vi "Get VS Channel Handles and Messages.vi"(8 "error in":errorcluster, 11 "custom device ref":T2 format="%.0x") -> (0 "error out":errorcluster, 1 "outgoing channels":T2[](array[typedef]) format="%.0x", 2 "incoming channels":T2[](array[typedef]) format="%.0x", 3 "custom device ref out":T2 format="%.0x", 4 "transmitted messages and subaddresses":T1[](array[typedef]) {"Timestamp Channel Handle" format="%.0x"; "Message Section Handle" format="%.0x"; "Parameter Channel Handles" format="%.0x"}, 6 "received messages and subaddresses":T1[](array[typedef]) {"Timestamp Channel Handle" format="%.0x"; "Message Section Handle" format="%.0x"; "Parameter Channel Handles" format="%.0x"})   [LabVIEW 2020, in "AIM MIL-STD-1553 Engine.lvlib" / "Implementation.lvlib" / "Execution Unit.lvclass"]
uses:
  Execution Unit.lvclass
  <vilib>/NI VeriStand/Custom Device API/Custom Device Item Ref.ctl
  Custom Device/Compiled Message.ctl
  Shared/Direction.ctl
  Shared/Parameter Definition.ctl
  <vilib>/NI VeriStand/Custom Device API/Custom Device API.lvlib
  Scripting/AIM MIL-STD-1553 Scripting.lvlib
  Custom Device/Custom Device.lvlib
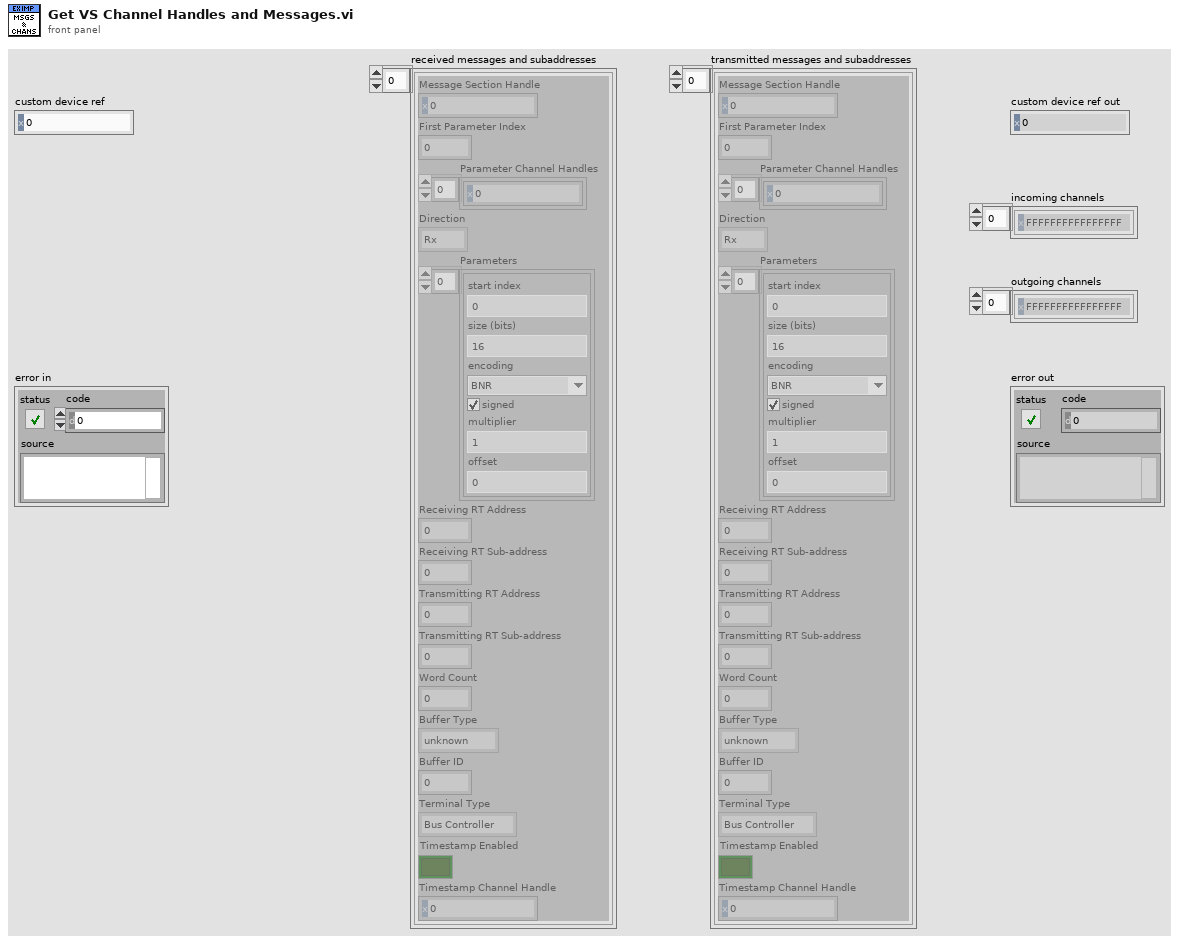
[diagram p1: front panel]
types:
  T1 = typedef "AIM MIL-STD-1553 Engine.lvlib/Custom Device.lvlib/Compiled Message.ctl" = cluster{"Message Section Handle":T2, "First Parameter Index":i32, "Parameter Channel Handles":T2[], "Direction":T3, "Parameters":T4[], "Receiving RT Address":u8, "Receiving RT Sub-address":u8, "Transmitting RT Address":u8, "Transmitting RT Sub-address":u8, "Word Count":u8, "Buffer Type":enum16{"unknown", "BC Message Buffer", "RT Message Buffer"}, "Buffer ID":u16, "Terminal Type":enum16{"Bus Controller", "Remote Terminal"}, "Timestamp Enabled":bool, "Timestamp Channel Handle":T2}
  T2 = typedef "Custom Device API.lvlib/Custom Device Item Ref.ctl" = u64
  T3 = typedef "Direction.ctl" = enum16{"Rx", "Tx"}
  T4 = typedef "Parameter Definition.ctl" = cluster{"start index":i32, "size (bits)":i32, "encoding":enum16{"BNR", "BCD", "Discrete"}, "signed":bool, "multiplier":dbl, "offset":dbl}
  T5 = typedef "Terminal Endpoint.ctl" = cluster{"terminal address":T6, "subaddress":T6}
  T6 = typedef "Address.ctl" = u16
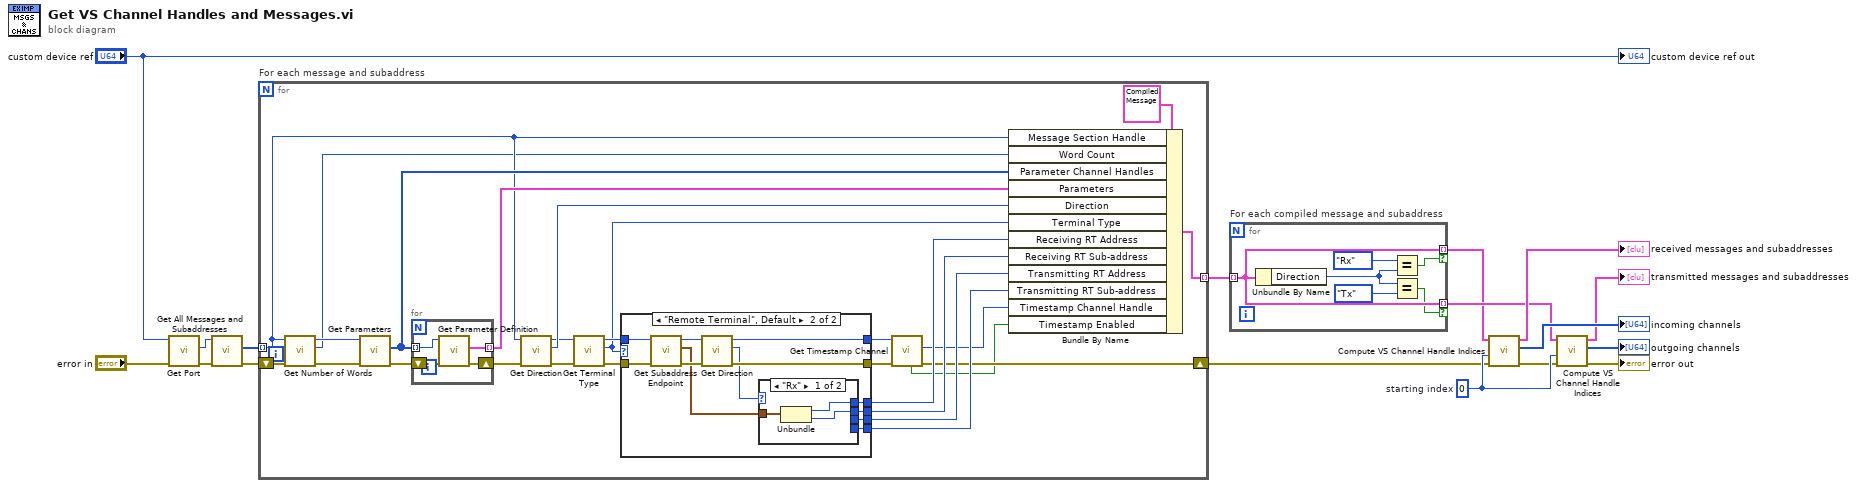
[diagram p0: block diagram]
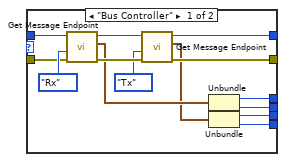
[diagram p2: hidden frame]
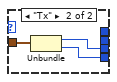
[diagram p3: hidden frame]
diagram:
  w12 = 0  # starting index
  n1 = call "Get Port.vi"("error in"="error in", "custom device ref"="custom device ref") -> ("error out"=w4:errorcluster, "port"=w3:T2)  [unwired: 6 in, 2 out]
  n2 = call "Get All Messages and Subaddresses.vi"("error in"=w4, "port"=w3) -> ("error out"=w11:errorcluster, "messages and subaddresses"=w10:T2[])  [unwired: 7 in, 1 out]
  n3 = for "For each message and subaddress" {
    shift-right: [w21] -> w6
    shift-left: w11 -> [w27]
    tunnel: w10 -> [w28] mode=indexing
    tunnel: [w43] -> w9 mode=indexing
    n4 = call "Get Number of Words.vi"("error in"=w27, "message or subaddress"=w28) -> ("error out"=w26:errorcluster, "number of words"=w24:u16, "message or subaddress out"=w25:T2)  [unwired: 7 in]
    n5 = call "Get Parameters.vi"("error in"=w26, "message or subaddress"=w25) -> ("error out"=w40:errorcluster, "parameters"=w39:T2[])  [unwired: 7 in, 1 out]
    n6 = for {
      shift-right: [w79] -> w37
      shift-left: w40 -> [w78]
      tunnel: w39 -> [w77] mode=indexing
      tunnel: [w76] -> w38 mode=indexing
      n7 = call "Get Parameter Definition.vi"("error in"=w78, "parameter"=w77) -> ("error out"=w79:errorcluster, "parameter definition"=w76:T4)  [unwired: 7 in, 1 out]
    }
    n8 = call "Get Direction.vi"("error in"=w37, "message or subaddress"=w28) -> ("error out"=w34:errorcluster, "direction"=w41:T3, "message or subaddress out"=w33:T2)  [unwired: 6 in, 1 out]
    n9 = call "Get Terminal Type.vi"("error in"=w34, "message or subaddress"=w33) -> ("error out"=w36:errorcluster, "terminal type"=w23:enum16{"Bus Controller", "Remote Terminal"}, "message or subaddress out"=w35:T2)  [unwired: 7 in]
    n10 = case shown="\"Remote Terminal\", Default" w23 {
      tunnel: [w51 w67] -> w20
      tunnel: [w50 w66] -> w22
      tunnel: w35 -> [w57 w63]
      tunnel: w36 -> [w55 w62]
      tunnel: [w44 w61] -> w29
      tunnel: [w45 w60] -> w30
      tunnel: [w48 w59] -> w31
      tunnel: [w49 w58] -> w32
      frame "Bus Controller" {
        n11 = call "Get Message Endpoint.vi"("error in"=w55, "direction"=Direction."Rx", "message"=w57) -> ("error out"=w54:errorcluster, "remote terminal endpoint"=w47:T5, "message out"=w52:T2)  [unwired: 5 in, 1 out]
        n12 = call "Get Message Endpoint.vi"("error in"=w54, "direction"=Direction."Tx", "message"=w52) -> ("error out"=w50:errorcluster, "remote terminal endpoint"=w46:T5, "message out"=w51:T2)  [unwired: 5 in, 1 out]
        n13 = Unbundle(w47) -> ("terminal address"=w49:T6, "subaddress"=w48:T6)
        n14 = Unbundle(w46) -> ("terminal address"=w45:T6, "subaddress"=w44:T6)
      }
      frame "Remote Terminal", Default {
        n15 = call "Get Subaddress Endpoint.vi"("error in"=w62, "subaddress"=w63) -> ("error out"=w68:errorcluster, "remote terminal endpoint"=w64:T5, "subaddress out"=w69:T2)  [unwired: 7 in]
        n16 = call "Get Direction.vi"("error in"=w68, "message or subaddress"=w69) -> ("error out"=w66:errorcluster, "direction"=w65:T3, "message or subaddress out"=w67:T2)  [unwired: 6 in, 1 out]
        n17 = case shown="\"Rx\"" w65 {
          tunnel: w64 -> [w72 w75]
          tunnel: [w71 _] -> w58
          tunnel: [w70 _] -> w59
          tunnel: [_ w74] -> w60
          tunnel: [_ w73] -> w61
          frame "Rx" {
            n18 = Unbundle(w72) -> ("terminal address"=w71:T6, "subaddress"=w70:T6)
          }
          frame "Tx" {
            n19 = Unbundle(w75) -> ("terminal address"=w74:T6, "subaddress"=w73:T6)
          }
        }
      }
    }
    n20 = call "Get Timestamp Channel.vi"("error in"=w22, "message section"=w20) -> ("error out"=w21:errorcluster, "timestamp channel"=w18:T2, "found?"=w19:bool)  [unwired: 6 in, 1 out]
    n21 = Bundle By Name(cluster=T1 {"Message Section Handle"=18446744073709551615, "First Parameter Index"=0, "Parameter Channel Handles"=[], "Direction"=enum."Rx", "Parameters"=[], "Receiving RT Address"=0, "Receiving RT Sub-address"=0, "Transmitting RT Address"=0, "Transmitting RT Sub-address"=0, "Word Count"=0, "Buffer Type"=enum."unknown", "Buffer ID"=0, "Terminal Type"=enum."Bus Controller", "Timestamp Enabled"=FALSE, "Timestamp Channel Handle"=0}, "Message Section Handle"=w28, "Word Count"=w24, "Parameter Channel Handles"=w39, "Parameters"=w38, "Direction"=w41, "Terminal Type"=w23, "Receiving RT Address"=w32, "Receiving RT Sub-address"=w31, "Transmitting RT Address"=w30, "Transmitting RT Sub-address"=w29, "Timestamp Channel Handle"=w18, "Timestamp Enabled"=w19) -> (w43:T1)
  }
  n22 = for "For each compiled message and subaddress" {
    tunnel: w9 -> [w85] mode=indexing
    tunnel: [w85] -> w7 mode=indexing if=w81
    tunnel: [w85] -> w8 mode=indexing if=w80
    n23 = Unbundle By Name(w85) -> ("Direction"=w84:T3)
    n24 = Equal?(x=Direction."Rx", y=w84) -> (x = y?=w81:bool)
    n25 = Equal?(x=w84, y=Direction."Tx" ("x")) -> (x = y?=w80:bool)
  }
  n26 = call "Compute VS Channel Handle Indices.vi"("error in (no error)"=w6, "next index"=w12, "messages and subaddresses"=w7) -> ("error out"=w5:errorcluster, "channel handles"=→"incoming channels":T2[], "messages and subaddresses out"=→"received messages and subaddresses":T1[])  [unwired: 5 in, 1 out]
  n27 = call "Compute VS Channel Handle Indices.vi"("error in (no error)"=w5, "next index"=w12, "messages and subaddresses"=w8) -> ("error out"=→"error out":errorcluster, "channel handles"=→"outgoing channels":T2[], "messages and subaddresses out"=→"transmitted messages and subaddresses":T1[])  [unwired: 5 in, 1 out]
  "custom device ref out" <- "custom device ref"
